vi "smartparking.vi"() -> ()   [LabVIEW 2014]
uses:
  <vilib>/MakerHub/LINX/Public/Peripherals/Digital/Digital Write 1 Chan.vi
  <vilib>/MakerHub/LINX/Public/Peripherals/Analog/Analog Read 1 Chan.vi
  <vilib>/MakerHub/LINX/Public/Peripherals/Digital/Digital Write N Chans.vi
  <vilib>/MakerHub/LINX/Public/Peripherals/Analog/Analog Read N Chans.vi
  <vilib>/MakerHub/LINX/Private/Local IO/LinxDigitalWrite.vi
  <vilib>/MakerHub/LINX/Public/Utilities/Check Channel.vi
  <vilib>/MakerHub/LINX/Private/Local IO/LinxAnalogRead.vi
  <vilib>/MakerHub/LINX/Public/Utilities/Open Serial.vi
  <vilib>/MakerHub/LINX/Public/Sensors/Motion/Servo/Servo Open One Channel.vi
  <vilib>/MakerHub/LINX/Private/Utilties/Generate Error.vi
  <vilib>/MakerHub/LINX/Public/Sensors/Motion/Servo/Servo Set Pulse Width One Channel.vi
  <vilib>/MakerHub/LINX/Public/Sensors/Motion/Servo/Servo Close One Channel.vi
  <vilib>/MakerHub/LINX/LMH-LINX.lvlib
  <vilib>/MakerHub/LINX/Public/Sensors/Motion/Servo/Servo.lvlib
panel:
  out "String":string
  out "Status:":string
  out "LDR 2":dbl
  out "LDR 1":dbl
  in  "Serial Port":refnum<visa-resource-name>="N/A"
  in  "stop":bool
  in  "Laser On/Off":bool=TRUE
  in  "jumlah parkir":dbl
  # "PARKIR TERSEDIA:"
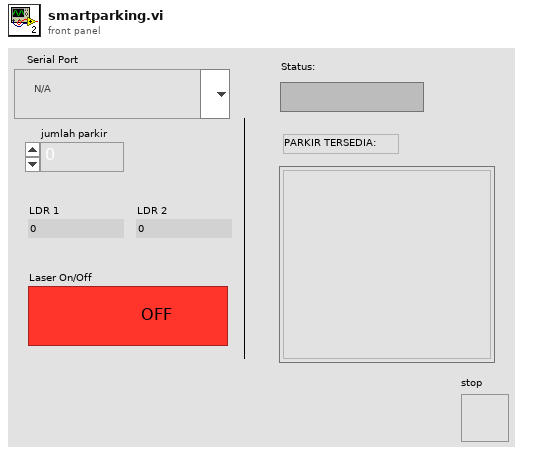
[diagram p1: front panel]
types:
  T1 = typedef "LMH-LINX.lvlib/LINX Ref.ctl" = cluster{"IO":T2, "Interface":T3, "LINX Device Config":T4}
  T2 = typedef "LMH-LINX.lvlib/Platform.ctl" = enum16{"Remote", "Local"}
  T3 = typedef "LMH-LINX.lvlib/Interface.ctl" = enum16{"Serial", "TCP"}
  T4 = typedef "LMH-LINX.lvlib/Device.lvlib/LINX Device Config.ctl" = cluster{"Interface":T3, "COM Port":refnum<visa-resource-name>, "TCP Configuration":T5, "Device Family":u8, "Device ID":u8, "Device Name":string, "TCP Ref":refnum<k5>, "Channels":T6}
  T5 = typedef "LMH-LINX.lvlib/Device.lvlib/TCP Config.ctl" = cluster{"IP Address":string, "Port":u16}
  T6 = typedef "LMH-LINX.lvlib/Channels.ctl" = cluster{"DI":u8[], "DO":u8[], "AI":u8[], "AO":u8[], "PWM":u8[], "QE":u8[], "UART":u8[], "I2C 2":u8[], "SPI":u8[], "CAN":u8[], "Servo":u8[], "AI Ref (V)":dbl, "AI Resolution (Bits)":u8, "AO Ref (V)":dbl, "AO Resolution (Bits)":u8}
  T7 = cluster{"0[0]":bool, "0[1]":bool, "0[2]":bool, "0[3]":bool, "0[4]":bool, "0[5]":bool, "0[6]":bool, "0[7]":bool, "0[8]":bool}
  T8 = cluster{"0 2[0]":bool, "0 2[1]":bool, "0 2[2]":bool, "0 2[3]":bool, "0 2[4]":bool, "0 2[5]":bool, "0 2[6]":bool, "0 2[7]":bool, "0 2[8]":bool}
  T9 = cluster{"0 3[0]":bool, "0 3[1]":bool, "0 3[2]":bool, "0 3[3]":bool, "0 3[4]":bool, "0 3[5]":bool, "0 3[6]":bool, "0 3[7]":bool, "0 3[8]":bool}
  T10 = cluster{"0 4[0]":bool, "0 4[1]":bool, "0 4[2]":bool, "0 4[3]":bool, "0 4[4]":bool, "0 4[5]":bool, "0 4[6]":bool, "0 4[7]":bool, "0 4[8]":bool}
  T11 = cluster{"0 5[0]":bool, "0 5[1]":bool, "0 5[2]":bool, "0 5[3]":bool, "0 5[4]":bool, "0 5[5]":bool, "0 5[6]":bool, "0 5[7]":bool, "0 5[8]":bool}
  T12 = cluster{"0 6[0]":bool, "0 6[1]":bool, "0 6[2]":bool, "0 6[3]":bool, "0 6[4]":bool, "0 6[5]":bool, "0 6[6]":bool, "0 6[7]":bool, "0 6[8]":bool}
  T13 = cluster{"0 7[0]":bool, "0 7[1]":bool, "0 7[2]":bool, "0 7[3]":bool, "0 7[4]":bool, "0 7[5]":bool, "0 7[6]":bool, "0 7[7]":bool, "0 7[8]":bool}
  T14 = cluster{"0 8[0]":bool, "0 8[1]":bool, "0 8[2]":bool, "0 8[3]":bool, "0 8[4]":bool, "0 8[5]":bool, "0 8[6]":bool, "0 8[7]":bool, "0 8[8]":bool}
  T15 = cluster{"0 9[0]":bool, "0 9[1]":bool, "0 9[2]":bool, "0 9[3]":bool, "0 9[4]":bool, "0 9[5]":bool, "0 9[6]":bool, "0 9[7]":bool, "0 9[8]":bool}
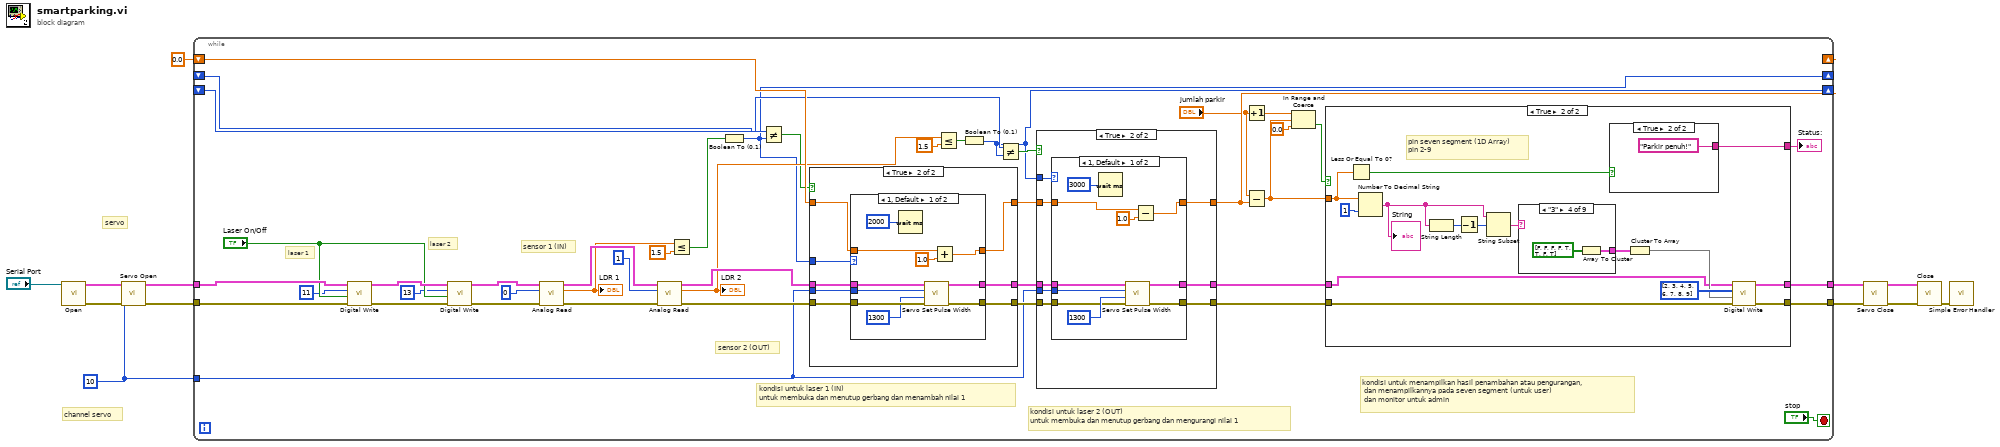
[diagram p0: block diagram]
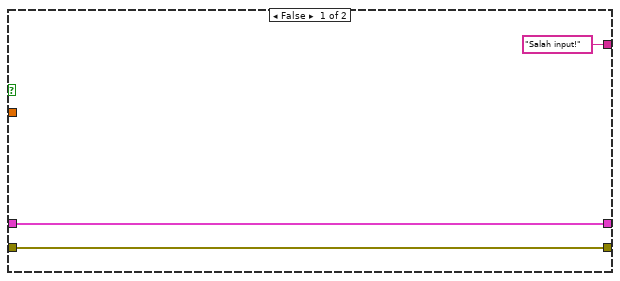
[diagram p2: hidden frame]
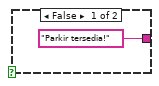
[diagram p3: hidden frame]
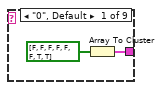
[diagram p4: hidden frame]
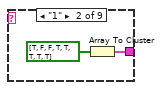
[diagram p5: hidden frame]
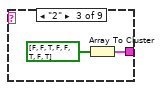
[diagram p6: hidden frame]
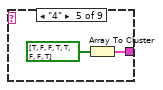
[diagram p7: hidden frame]
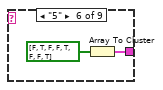
[diagram p8: hidden frame]
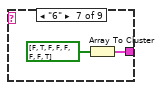
[diagram p9: hidden frame]
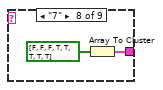
[diagram p10: hidden frame]
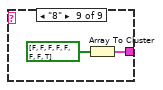
[diagram p11: hidden frame]
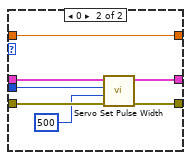
[diagram p13: hidden frame]
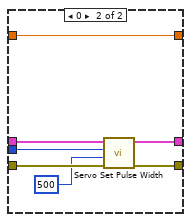
[diagram p15: hidden frame]
diagram:
  w1 = u8 10 ("Servo Channel")
  # "channel servo"
  # "servo"
  n1 = call-poly <vilib>:"Open.vi"("Serial Port"="Serial Port") -> ("Error Out"=w9:errorcluster, "LINX Resource"=w10:T1)  [unwired: 8 in, 1 out]
  n2 = call-poly <vilib>:"Servo Open.vi"("Error In"=w9, "Servo Channel"=w1, "LINX Resource"=w10) -> ("Error Out"=w7:errorcluster, "LINX Resource"=w8:T1)  [unwired: 7 in]
  n3 = while {
    tunnel: [w22] -> w6
    tunnel: w8 -> [w55]
    tunnel: [w21] -> w5
    tunnel: w7 -> [w54]
    shift-right: [w53] -> _
    shift-left: 0.0 ("x") -> [w46]
    shift-right: [w15] -> _
    shift-left: _ -> [w45]
    shift-right: [w14] -> _
    shift-left: _ -> [w44]
    tunnel: w1 -> [w13]
    stop <- "stop" stop-if-true
    # "kondisi untuk menampilkan hasil penambahan atau pengurangan,\n dan menampilkannya pada seven segment (untuk user)\n dan monitor untuk admin"
    # "kondisi untuk laser 2 (OUT)\nuntuk membuka dan menutup gerbang dan mengurangi nilai 1"
    # "kondisi untuk laser 1 (IN)\nuntuk membuka dan menutup gerbang dan menambah nilai 1"
    # "sensor 2 (OUT)"
    # "sensor 1 (IN)"
    # "laser 2"
    # "laser 1"
    n4 = call-poly <vilib>:"Digital Write.vi"("Error In"=w54, "Output Value"="Laser On/Off", "DO Channel"=u8 11, "LINX Resource"=w55) -> ("Error Out"=w51:errorcluster, "LINX Resource"=w52:T1)  [unwired: 6 in]
    n5 = call-poly <vilib>:"Digital Write.vi"("Error In"=w51, "Output Value"="Laser On/Off", "DO Channel"=u8 13, "LINX Resource"=w52) -> ("Error Out"=w40:errorcluster, "LINX Resource"=w41:T1)  [unwired: 6 in]
    n6 = call-poly <vilib>:"Analog Read.vi"("Error In"=w40, "Analog Channel"=u8 0 ("pin sensor 1"), "LINX Resource"=w41) -> ("Error Out"=w38:errorcluster, "Voltage"=w35:dbl, "LINX Resource"=w39:T1)  [unwired: 5 in, 1 out]
    "LDR 1" <- w35
    n7 = call-poly <vilib>:"Analog Read.vi"("Error In"=w38, "Analog Channel"=u8 1 ("pin sensor 2"), "LINX Resource"=w39) -> ("Error Out"=w36:errorcluster, "Voltage"=w28:dbl, "LINX Resource"=w37:T1)  [unwired: 5 in, 1 out]
    "LDR 2" <- w28
    n8 = Less Or Equal?(x=w35, y=1.5) -> (x <= y?=w33:bool)
    n9 = Boolean To (0,1)(Boolean=w33) -> (0, 1=w15:i16)
    n10 = Not Equal?(x=w45, y=w15) -> (x != y?=w17:bool)
    n11 = case shown="True" w17 {
      tunnel: [w97 w105] -> w49
      tunnel: [w96 w104] -> w48
      tunnel: [w95 w103] -> w47
      tunnel: w36 -> [w95 w102]
      tunnel: w37 -> [w96 w101]
      tunnel: w46 -> [w97 w100]
      tunnel: w15 -> [_ w99]
      tunnel: w13 -> [_ w98]
      frame False {
      }
      frame True {
        n12 = case shown="1, Default" w99 {
          tunnel: w100 -> [w108 w117]
          tunnel: [w109 w117] -> w105
          tunnel: w101 -> [w115 w122]
          tunnel: w102 -> [w114 w121]
          tunnel: [w112 w120] -> w104
          tunnel: [w111 w119] -> w103
          tunnel: w98 -> [w106 w116]
          frame 1, Default {
            n13 = Wait (ms)(milliseconds to wait=u32 2000) -> ()  [unwired: 1 out]
            n14 = call-poly <vilib>:"Servo Set Pulse Width.vi"("Error In"=w114, "Pulse Width (uS)"=u16 1300, "Servo Channel"=w106, "LINX Resource"=w115) -> ("Error Out"=w111:errorcluster, "LINX Resource"=w112:T1)  [unwired: 6 in]
            n15 = Add(x=w108, y=1.0) -> (x+y=w109:dbl)
          }
          frame 0 {
            n16 = call-poly <vilib>:"Servo Set Pulse Width.vi"("Error In"=w121, "Pulse Width (uS)"=u16 500, "Servo Channel"=w116, "LINX Resource"=w122) -> ("Error Out"=w119:errorcluster, "LINX Resource"=w120:T1)  [unwired: 6 in]
          }
        }
      }
    }
    n17 = Less Or Equal?(x=w28, y=1.5) -> (x <= y?=w29:bool)
    n18 = Boolean To (0,1)(Boolean=w29) -> (0, 1=w14:i16)
    n19 = Not Equal?(x=w44, y=w14) -> (x != y?=w16:bool)
    n20 = case shown="True" w16 {
      tunnel: w49 -> [w125 w129]
      tunnel: [w125 w128] -> w53
      tunnel: w48 -> [w124 w133]
      tunnel: w47 -> [w123 w132]
      tunnel: [w124 w131] -> w23
      tunnel: [w123 w130] -> w24
      tunnel: w14 -> [_ w127]
      tunnel: w13 -> [_ w126]
      frame False {
      }
      frame True {
        n21 = case shown="1, Default" w127 {
          tunnel: w133 -> [w139 w150]
          tunnel: w132 -> [w138 w149]
          tunnel: [w137 w148] -> w131
          tunnel: [w136 w147] -> w130
          tunnel: w129 -> [w141 w145]
          tunnel: [w140 w145] -> w128
          tunnel: w126 -> [w134 w144]
          frame 1, Default {
            n22 = Wait (ms)(milliseconds to wait=u32 3000) -> ()  [unwired: 1 out]
            n23 = call-poly <vilib>:"Servo Set Pulse Width.vi"("Error In"=w138, "Pulse Width (uS)"=u16 1300, "Servo Channel"=w134, "LINX Resource"=w139) -> ("Error Out"=w136:errorcluster, "LINX Resource"=w137:T1)  [unwired: 6 in]
            n24 = Subtract(x=w141, y=1.0) -> (x-y=w140:dbl)
          }
          frame 0 {
            n25 = call-poly <vilib>:"Servo Set Pulse Width.vi"("Error In"=w149, "Pulse Width (uS)"=u16 500, "Servo Channel"=w144, "LINX Resource"=w150) -> ("Error Out"=w147:errorcluster, "LINX Resource"=w148:T1)  [unwired: 6 in]
          }
        }
      }
    }
    n26 = Increment(x="jumlah parkir") -> (x+1=w19:dbl)
    n27 = Subtract(x="jumlah parkir", y=w53) -> (x-y=w25:dbl)
    n28 = In Range and Coerce(upper limit=w19, x=w25, lower limit=0.0) -> (In Range?=w26:bool)  [unwired: 1 out]
    n29 = case shown="True" w26 {
      tunnel: w25 -> [_ w62]
      tunnel: w24 -> [w58 w66]
      tunnel: w23 -> [w59 w65]
      tunnel: [w59 w64] -> w22
      tunnel: [w58 w63] -> w21
      tunnel: ["Salah input!" ("Status:") w61] -> w20
      frame False {
      }
      frame True {
        # "pin seven segment (1D Array)\npin 2-9"
        n30 = Less Or Equal To 0?(x=w62) -> (x <= 0?=w67:bool)
        n31 = Number To Decimal String(number=w62, width (-)=i16 1) -> (decimal integer string=w60:string)
        "String" <- w60
        n32 = String Length(string=w60) -> (length=w74:i32)
        n33 = Decrement(x=w74) -> (x-1=w73:i32)
        n34 = String Subset(string=w60, offset (0)=w73) -> (substring=w70:string)  [unwired: 1 in]
        n35 = case shown="\"3\"" w70 {
          tunnel: [w77 w79 w81 w83 w85 w87 w89 w91 w93] -> w69
          frame "0", Default {
            n36 = Array To Cluster(array=bool[] [FALSE, FALSE, FALSE, FALSE, FALSE, FALSE, TRUE, TRUE] ("0")) -> (cluster=w77:T7)
          }
          frame "1" {
            n37 = Array To Cluster(array=bool[] [TRUE, FALSE, FALSE, TRUE, TRUE, TRUE, TRUE, TRUE] ("0 2")) -> (cluster=w79:T8)
          }
          frame "2" {
            n38 = Array To Cluster(array=bool[] [FALSE, FALSE, TRUE, FALSE, FALSE, TRUE, FALSE, TRUE] ("0 3")) -> (cluster=w81:T9)
          }
          frame "3" {
            n39 = Array To Cluster(array=bool[] [FALSE, FALSE, FALSE, FALSE, TRUE, TRUE, FALSE, TRUE] ("0 4")) -> (cluster=w83:T10)
          }
          frame "4" {
            n40 = Array To Cluster(array=bool[] [TRUE, FALSE, FALSE, TRUE, TRUE, FALSE, FALSE, TRUE] ("0 5")) -> (cluster=w85:T11)
          }
          frame "5" {
            n41 = Array To Cluster(array=bool[] [FALSE, TRUE, FALSE, FALSE, TRUE, FALSE, FALSE, TRUE] ("0 6")) -> (cluster=w87:T12)
          }
          frame "6" {
            n42 = Array To Cluster(array=bool[] [FALSE, TRUE, FALSE, FALSE, FALSE, FALSE, FALSE, TRUE] ("0 7")) -> (cluster=w89:T13)
          }
          frame "7" {
            n43 = Array To Cluster(array=bool[] [FALSE, FALSE, FALSE, TRUE, TRUE, TRUE, TRUE, TRUE] ("0 8")) -> (cluster=w91:T14)
          }
          frame "8" {
            n44 = Array To Cluster(array=bool[] [FALSE, FALSE, FALSE, FALSE, FALSE, FALSE, FALSE, TRUE] ("0 9")) -> (cluster=w93:T15)
          }
        }
        n45 = case shown="True" w67 {
          tunnel: ["Parkir tersedia!" ("Status:") "Parkir penuh!" ("Status:")] -> w61
          frame False {
          }
          frame True {
          }
        }
        n46 = Cluster To Array(cluster=w69) -> (array=w68:bool[])
        n47 = call-poly <vilib>:"Digital Write.vi"("Error In"=w66, "Values"=w68, "DO Channels"=u8[] [2, 3, 4, 5, 6, 7, 8, 9], "LINX Resource"=w65) -> ("Error Out"=w63:errorcluster, "LINX Resource"=w64:T1)  [unwired: 6 in]
      }
    }
    "Status:" <- w20
  }
  n48 = call-poly <vilib>:"Servo Close.vi"("Error In"=w5, "LINX Resource"=w6) -> ("Error Out"=w3:errorcluster, "LINX Resource"=w4:T1)  [unwired: 8 in]
  n49 = call <vilib>:"Close.vi"("Error In"=w3, "LINX Resource"=w4) -> ("Error Out"=w2:errorcluster)  [unwired: 9 in]
  n50 = call <vilib>:"Simple Error Handler.vi"("error in (no error)"=w2) -> ()  [unwired: 4 in, 5 out]
